vi "pid-toolkit-control.vi"() -> ()   [LabVIEW 2018, in "pid-toolkit.lvlib"]
uses:
  pid-toolkit.lvlib
  <vilib>/Platform/TimedLoop/XDataNode/timing_clust.ctl
  <vilib>/Platform/TimedLoop/XDataNode/nitl_modes.ctl
  <vilib>/Platform/TimedLoop/XDataNode/wakeup.ctl
  <vilib>/platform/TimedLoop/XDataNode/XDataNode.xnode
  <vilib>/Platform/TimedLoop/XDataNode/XDNodeRunTimeDep.lvlib
panel:
  out "TDMS error":errorcluster
  in  "Log to TDMS file":bool
  out "TDMS Path":path
  in  "Clear Error":bool
  in  "Refresh Button":bool
  out "Measurments":dbl[](array[numeric])
  in  "Down Button":bool
  in  "Manual":dbl(slide) scale=0.0..255.0
  out "Output":u16(knob) scale=0.0..255.0 scale format="%x"
  in  "KdTd":sgl caption="Kd"
  in  "KiTi":sgl caption="Ki"
  in  "Kp":sgl
  out "PID Integral":sgl
  out "PID Error":sgl
  out "PID Derivative":sgl
  in  "Automatic":bool=TRUE
  out "output range":cluster{"output high":dbl, "output low":dbl}={"output high"=100.0, "output low"=-100.0} {"output low" format="%.2f"; "output high" format="%.2f"}
  out "Plot":T1(graph)
  in  "Setpoint":dbl(slide) scale=0.0..300.0
  out "Modbus error":errorcluster
  in  "Off Hook":bool
  in  "Update Rate":dbl caption="Rate"
  out "Failure":bool
  out "Updating":bool
  in  "Update Now":bool
  in  "Maximum":sgl
  in  "Minimum":sgl
  out "Thermometer":sgl(slide) scale=0.0..260.0
  in  "Force exit out of loop":bool
  out "Interval":i64
  out "Duration":i64
  out "Cycle":i32
  in  "Frequency":dbl(slide) scale=0.1..10.0
  # "Loop"
  # "Modbus"
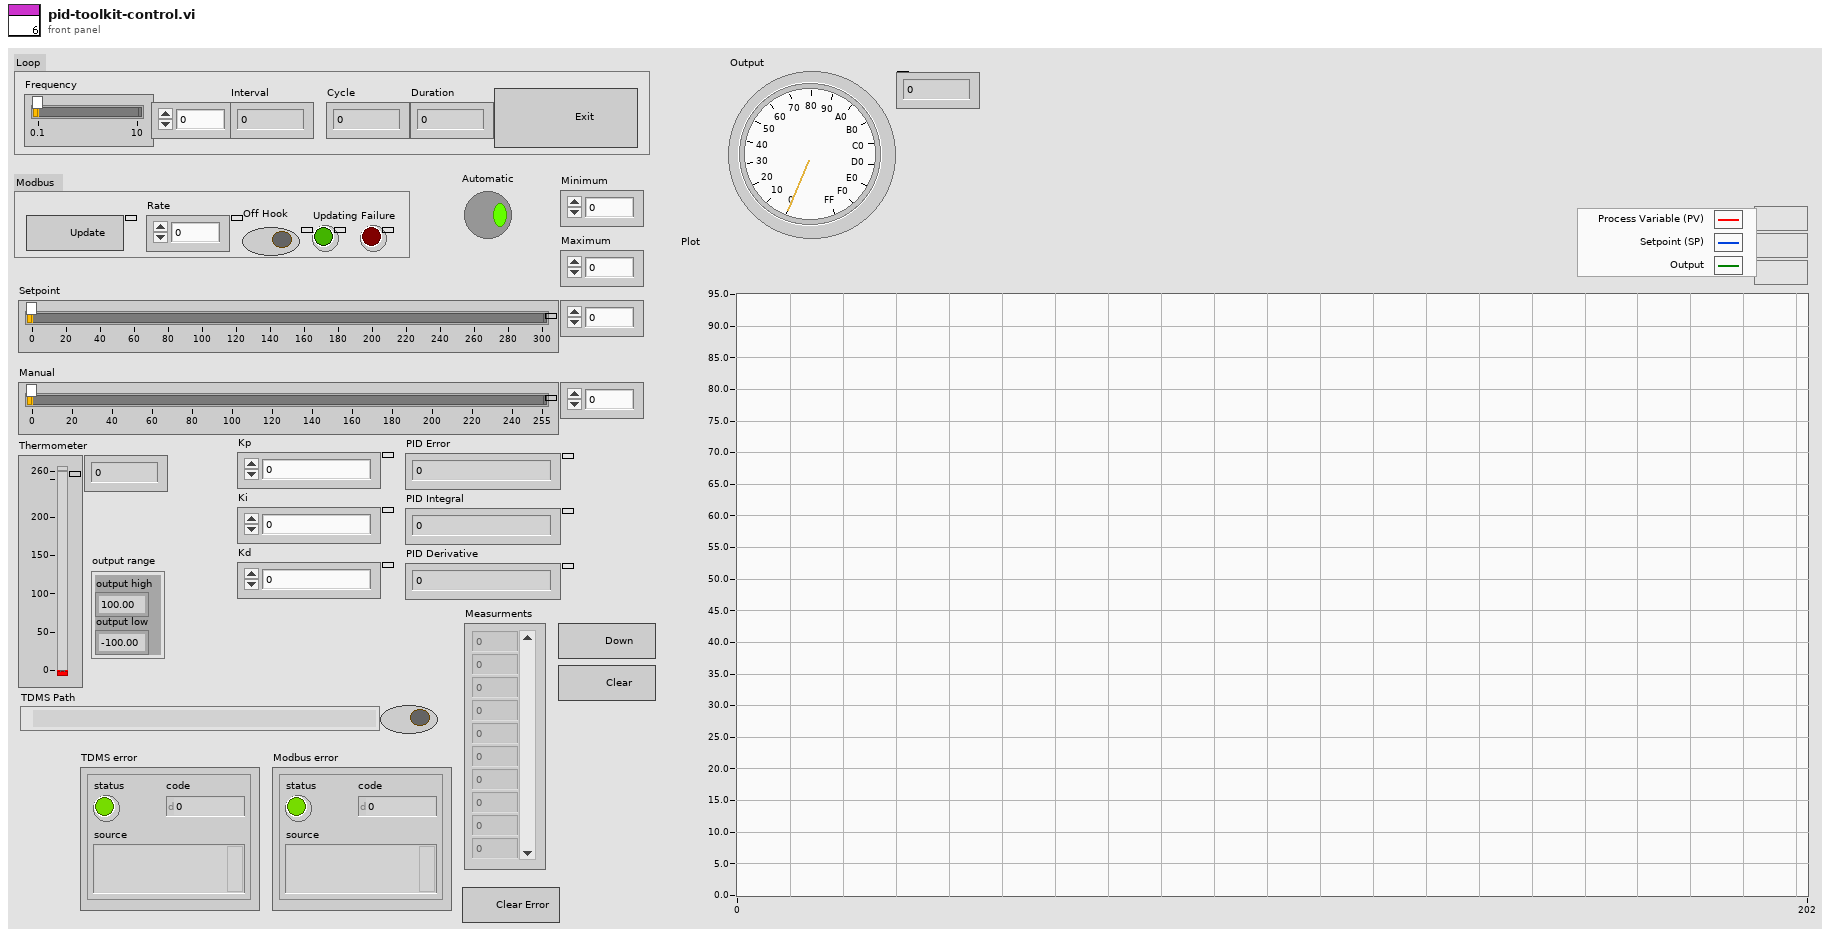
[diagram p1: front panel]
types:
  T1 = cluster{dbl, "desired temperature":dbl, "output":dbl}
  T2 = enum16{"open", "open or create", "create or replace", "create", "open (read-only)"}
  T3 = typedef "XDNodeRunTimeDep.lvlib/timing_clust.ctl" = cluster{"Expected End [f-1]":u64, "Actual End [f-1]":u64, "Finished Late? [f-1]":bool, "Expected End [i-1]":u64, "Actual End [i-1]":u64, "Finished Late? [i-1]":bool, "Expected Start [i]":u64, "Actual Start [i]":u64, "Expected Start [f]":u64, "Actual Start [f]":u64, "Source Name":string, "Structure Name":string, "Period":i64, "Deadline":i64, "Offset":i64, "Start":i64, "Priority":i32, "Timeout":i32, "Mode":T4, "Wakeup Reason":T5, "Error":errorcluster, "Source Type":string, "Secondary Source Type":string, "Global End Time":u64, "Global Start Time":u64, "Frame Duration":u64, "Iteration Duration":u64, "Assigned CPU":i32, "I/O Scan Engine Mode":u32}
  T4 = typedef "XDNodeRunTimeDep.lvlib/nitl_modes.ctl" = enum32{"No Change", "Process missed periods, maintain original phase", "Discard missed periods, maintain original phase", "Process missed periods, ignore original phase", "Discard missed periods, ignore original phase"}
  T5 = typedef "XDNodeRunTimeDep.lvlib/wakeup.ctl" = enum32{"Normal", "Aborted", "Asynchronous wakeup", "Timing source error", "Timed loop error", "Timeout"}
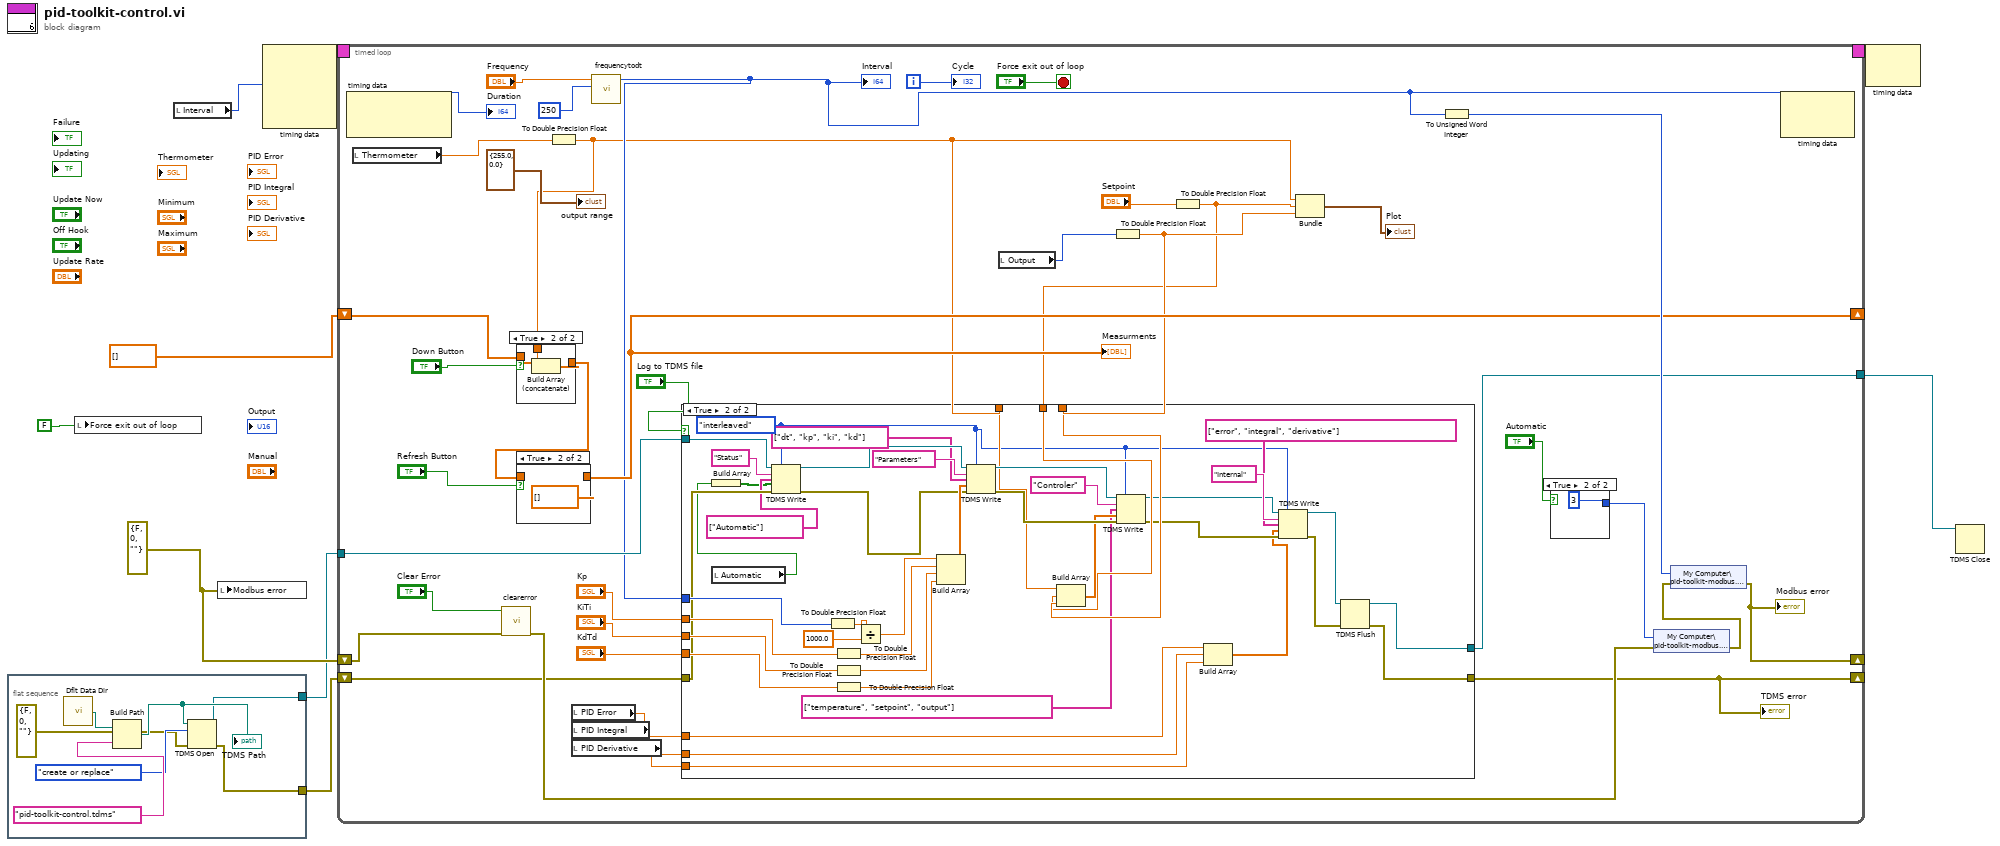
[diagram p0: block diagram]
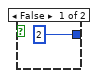
[diagram p5: hidden frame]
diagram:
  w5 = errorcluster {"status"=FALSE, "code"=0, "source"=""} ("Modbus error")
  n1 = flat-sequence {
    tunnel: [w11] -> w3
    tunnel: [w10] -> w1
    frame #0 {
      n2 = call <vilib>:"Dflt Data Dir.vi"() -> ("App:Default Data Directory"=w16:path)
      n3 = Build Path(base path=w16, name or relative path="pid-toolkit-control.tdms") -> (appended path=w14:path)
      "TDMS Path" <- w14
      n4 = TDMS Open(8:errorcluster {"status"=FALSE, "code"=0, "source"=""} ("Modbus error"), 10:T2."create or replace" ("operation (0:open)"), 11:w14) -> (0:w10:errorcluster, 3:w11:refnum<k34>)  [unwired: 4 in]
    }
  }
  n5 = local write "Force exit out of loop"(FALSE ("Force exit out of loop")) -> ()
  n6 = local read "Interval"() -> (w6:i64)
  n7 = local write "Modbus error"(w5) -> ()
  n8 = node-c288(w6) -> (w9:T3)  [unwired: 3 in]
  n9 = timed-loop {
    timing: w9 -> [_]
    timing-out: [_] -> w8
    shift-right: [w45] -> _
    shift-left: w5 -> [w35]
    shift-right: [w37] -> _
    shift-left: dbl[] [] ("Measurments") -> [w39]
    tunnel: w3 -> [w30]
    tunnel: [w29] -> w2
    shift-right: [w20] -> _
    shift-left: w1 -> [w28]
    i -> [w50]
    stop <- "Force exit out of loop" stop-if-true
    n10 = node-c288() -> (→"Duration":i64)  [unwired: 1 in, 1 out]
    n11 = local read "Thermometer"() -> (w48:sgl)
    n12 = call "clearerror.vi"("error in (no error)"=w35, "Clear Error"="Clear Error") -> ("error out"=w34:errorcluster)  [unwired: 9 in]
    n13 = To Double Precision Float(number=w48) -> (double precision float=w21:dbl)
    n14 = case shown="True" "Down Button" {
      tunnel: w21 -> [_ w104]
      tunnel: w39 -> [w101 w103]
      tunnel: [w101 w102] -> w36
      frame False {
      }
      frame True {
        n15 = Build Array (concatenate)(w103, w104) -> (w102:dbl[])
      }
    }
    n16 = case shown="True" "Refresh Button" {
      tunnel: [w99 dbl[] [] ("Measurments")] -> w37
      tunnel: w36 -> [w99 _]
      frame False {
      }
      frame True {
      }
    }
    "Measurments" <- w37
    n17 = local read "PID Error"() -> (w19:sgl)
    n18 = local read "PID Integral"() -> (w18:sgl)
    n19 = local read "PID Derivative"() -> (w17:sgl)
    n20 = call "frequencytodt.vi"("Default in"=i64 250, "Frequency"="Frequency") -> ("Default out"=w27:i64)  [unwired: 9 in]
    "Interval" <- w27
    n21 = local read "Output"() -> (w43:u16)
    n22 = To Double Precision Float(number=w43) -> (double precision float=w23:dbl)
    n23 = To Double Precision Float(number="Setpoint") -> (double precision float=w22:dbl)
    n24 = case shown="True" "Log to TDMS file" {
      tunnel: w30 -> [w56 w68]
      tunnel: [w56 w97] -> w29
      tunnel: w28 -> [w55 w65]
      tunnel: [w55 w95] -> w20
      tunnel: w27 -> [_ w93]
      tunnel: "Kp" -> [_ w89]
      tunnel: "KiTi" -> [_ w88]
      tunnel: "KdTd" -> [_ w87]
      tunnel: w23 -> [_ w79]
      tunnel: w22 -> [_ w78]
      tunnel: w21 -> [_ w81]
      tunnel: w19 -> [_ w72]
      tunnel: w18 -> [_ w71]
      tunnel: w17 -> [_ w70]
      frame False {
      }
      frame True {
        w57 = enum16{"decimated", "interleaved"}."interleaved" ("data layout (0:decimated)")
        n25 = local read "Automatic"() -> (w62:bool)
        n26 = Build Array(w62) -> (w61:bool[])
        n27 = TDMS Write(0:w68, 1:w57, 5:"Status" ("group name in (Untitled)"), 7:string[] ["Automatic"] ("channel name(s) in (Untitled)"), 9:w61, 11:w65) -> (4:w66:refnum<k34>, 15:w64:errorcluster)  [unwired: 2 out]
        n28 = To Double Precision Float(number=w93) -> (double precision float=w92:dbl)
        n29 = To Double Precision Float(number=w89) -> (double precision float=w86:dbl)
        n30 = To Double Precision Float(number=w88) -> (double precision float=w85:dbl)
        n31 = To Double Precision Float(number=w87) -> (double precision float=w84:dbl)
        n32 = Divide(x=w92, y=1000.0) -> (x/y=w90:dbl)
        n33 = Build Array(w90, w86, w85, w84) -> (w94:dbl[])
        n34 = TDMS Write(0:w66, 1:w57, 5:"Parameters" ("group name in (Untitled)"), 7:string[] ["dt", "kp", "ki", "kd"] ("channel name(s) in (Untitled)"), 9:w94, 11:w64) -> (4:w83:refnum<k34>, 15:w96:errorcluster)  [unwired: 2 out]
        n35 = Build Array(w81, w78, w79) -> (w80:dbl[])
        n36 = TDMS Write(0:w83, 1:w57, 5:"Controler" ("group name in (Untitled)"), 7:string[] ["temperature", "setpoint", "output"] ("channel name(s) in (Untitled)"), 9:w80, 11:w96) -> (4:w76:refnum<k34>, 15:w75:errorcluster)  [unwired: 2 out]
        n37 = Build Array(w72, w71, w70) -> (w69:sgl[])
        n38 = TDMS Write(0:w76, 1:w57, 5:"Internal" ("group name in (Untitled)"), 7:string[] ["error", "integral", "derivative"] ("channel name(s) in (Untitled)"), 9:w69, 11:w75) -> (4:w73:refnum<k34>, 15:w74:errorcluster)  [unwired: 2 out]
        n39 = TDMS Flush(4:w74, 7:w73) -> (0:w95:errorcluster, 3:w97:refnum<k34>)
      }
    }
    "TDMS error" <- w20
    n40 = Bundle(w21, w22, w23) -> (→"Plot":cluster{dbl, dbl, dbl})  [unwired: 1 in]
    n41 = To Unsigned Word Integer(number=w27) -> (unsigned 16bit integer=w49:u16)
    n42 = case shown="True" "Automatic" {
      tunnel: [u16 2 ("400016") u16 3 ("400016")] -> w41
      frame False {
      }
      frame True {
      }
    }
    n43 = shared-variable "My Computer\\pid-toolkit-modbus.lvlib\\400016"(w41, error in=w34) -> (error out=w42:errorcluster)
    n44 = shared-variable "My Computer\\pid-toolkit-modbus.lvlib\\400001"(w49, error in=w42) -> (error out=w45:errorcluster)
    "Modbus error" <- w45
    n45 = node-c288(w27) -> ()  [unwired: 1 in, 1 out]
    "Cycle" <- w50
    "output range" <- cluster{"output high":dbl, "output low":dbl} {"output high"=255.0, "output low"=0.0} ("output range")
  }
  n46 = node-c288(w8) -> ()  [unwired: 1 out]
  n47 = TDMS Close(11:w2) -> ()  [unwired: 1 in, 2 out]
